vi "Convert4ByteToInt.vi"(1 "Input":string="ÝÌ»ª") -> (0 "Output":u32 format="%.0x")   [LabVIEW 2019]
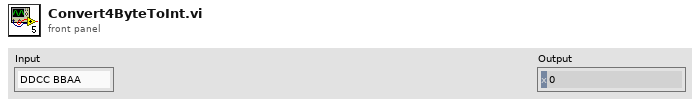
[diagram p1: front panel]
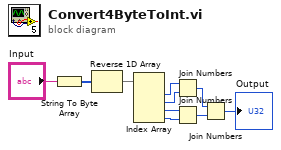
[diagram p0: block diagram]
diagram:
  n1 = String To Byte Array(string="Input") -> (unsigned byte array=w3:u8[])
  n2 = Reverse 1D Array(array=w3) -> (reversed array=w9:u8[])
  n3 = Index Array(array=w9) -> (element #1=w8:u8, element #2=w7:u8, element #3=w6:u8, element #4=w1:u8)  [unwired: 4 in]
  n4 = Join Numbers(hi=w8, lo=w7) -> ((hi.lo)=w5:u16)
  n5 = Join Numbers(hi=w6, lo=w1) -> ((hi.lo)=w4:u16)
  n6 = Join Numbers(hi=w5, lo=w4) -> ((hi.lo)=→"Output":u32)
